vi "SetParamWaveCommonPhase.vi"(1 "Selection":u16(ring) items=["Value", "Default", "Minimum", "Maximum"], 3 "error in (no error)":errorcluster, 4 "Phase [°]":u32, 5 "ParamWave Name":string, 6 "VISA resource name":refnum<visa-resource-name>) -> (0 "error out":errorcluster, 2 "VISA resource name out":refnum<visa-resource-name>)   [LabVIEW 2020, in "Active Technologies AWG3000.lvlib"]
uses:
  Active Technologies AWG3000.lvlib
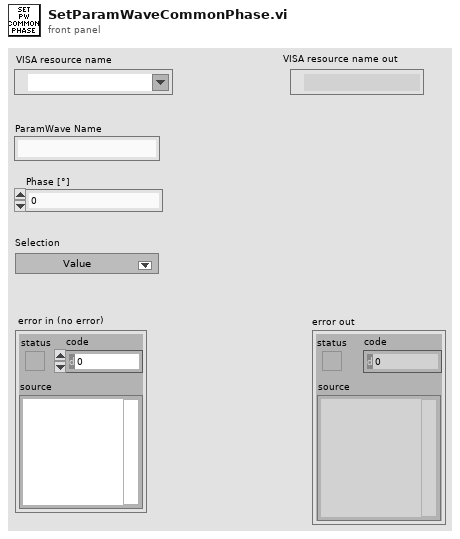
[diagram p1: front panel]
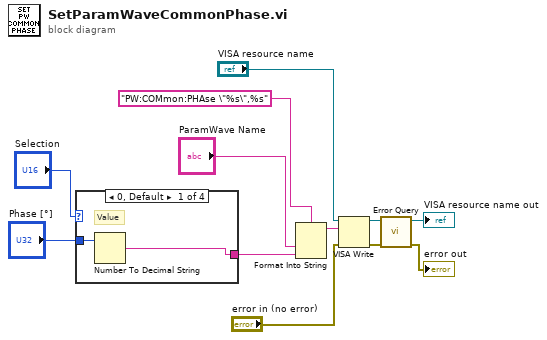
[diagram p0: block diagram]
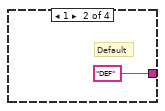
[diagram p2: hidden frame]
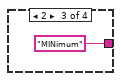
[diagram p3: hidden frame]
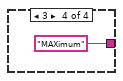
[diagram p4: hidden frame]
diagram:
  n1 = case shown="0, Default" "Selection" {
    tunnel: [w14 "DEF" ("write buffer") "MINimum" ("write buffer") "MAXimum" ("write buffer")] -> w2
    tunnel: "Phase [°]" -> [w13 _ _ _]
    frame 0, Default {
      # "Value"
      n2 = Number To Decimal String(number=w13) -> (decimal integer string=w14:string)  [unwired: 1 in]
    }
    frame 1 {
      # "Default"
    }
    frame 2 {
    }
    frame 3 {
    }
  }
  n3 = Format Into String(format string="PW:COMmon:PHAse \"%s\",%s" ("write buffer"), "ParamWave Name", w2) -> (resulting string=w1:string)  [unwired: 2 in, 1 out]
  n4 = VISA Write(VISA resource name="VISA resource name", write buffer=w1, error in (no error)="error in (no error)") -> (VISA resource name out=w10:refnum<visa-resource-name>, error out=w9:errorcluster)  [unwired: 1 out]
  n5 = call "Error Query.vi"("error in (no error)"=w9, "VISA resource name"=w10) -> ("error out"=→"error out":errorcluster, "VISA resource name out"=→"VISA resource name out":refnum<visa-resource-name>)  [unwired: 6 in, 2 out]
